vi "subBuildAppRelativePath.vi"(10 "String path":string, 11 "App path":path) -> (3 "appended path":path)   [LabVIEW 2020, in "CommonHelpers.lvlib"]
uses:
  CommonHelpers.lvlib
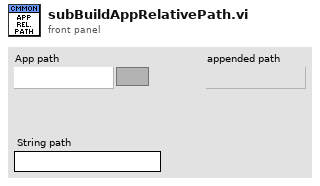
[diagram p1: front panel]
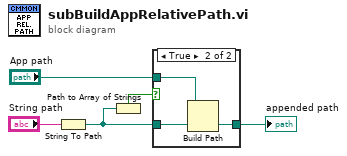
[diagram p0: block diagram]
diagram:
  n1 = String To Path(string="String path") -> (path=w2:path)
  n2 = Path to Array of Strings(0:w2) -> (1:w1:bool)  [unwired: 1 out]
  n3 = case shown="True" w1 {
    tunnel: w2 -> [w6 w8]
    tunnel: "App path" -> [_ w9]
    tunnel: [w6 w7] -> w4
    frame False {
    }
    frame True {
      n4 = Build Path(base path=w9, name or relative path=w8) -> (appended path=w7:path)
    }
  }
  "appended path" <- w4
